vi "Transmit Command.vi"(8 "error in":errorcluster, 10 "Command":string, 11 "3300 in":refnum<class "3300.lvclass">) -> (0 "error out":errorcluster, 3 "3300 out":refnum<class "3300.lvclass">)   [LabVIEW 2019, in "3300.lvlib" / "3300.lvclass"]
uses:
  Library/3300.lvclass
  Library/3300.lvclass/3300.ctl
  <instrlib>/Agilent N330X Series/Agilent N330X Series.lvlib
  builds/Engine/Engine.lvlibp/Project/Engine.lvclass
  C:/Users/Public/Documents/Development/builds/Engine/Engine.lvlibp/Project/Engine.lvclass
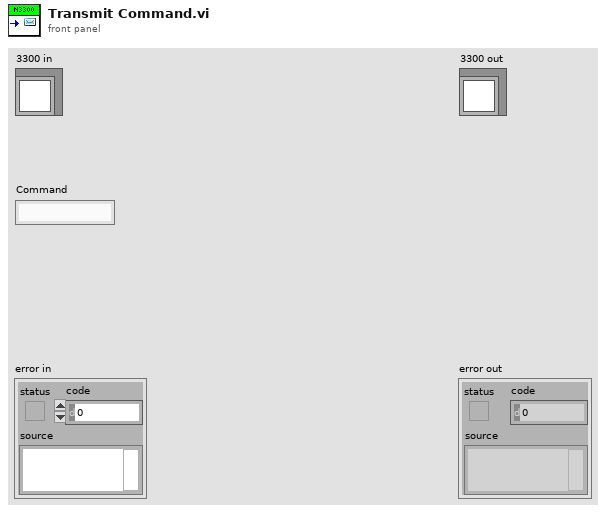
[diagram p1: front panel]
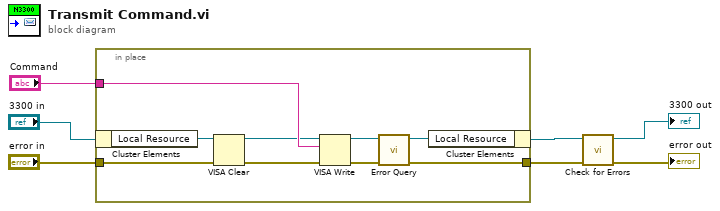
[diagram p0: block diagram]
diagram:
  n1 = in-place {
    in-place-border: "Command" -> [w15]
    in-place-border: "error in" -> [w8]
    in-place-border: [w11] -> w3
    n2 = in-place-cluster #1("3300 in") -> ("Local Resource"=w16:refnum<visa-resource-name>)
    n3 = VISA Clear(VISA resource name=w16, error in (no error)=w8) -> (VISA resource name out=w10:refnum<visa-resource-name>, error out=w9:errorcluster)
    n4 = VISA Write(VISA resource name=w10, write buffer=w15, error in (no error)=w9) -> (VISA resource name out=w14:refnum<visa-resource-name>, error out=w13:errorcluster)  [unwired: 1 out]
    n5 = call <instrlib>:"Error Query.vi"("error in (no error)"=w13, "VISA resource name"=w14) -> ("error out"=w11:errorcluster, "VISA resource name out"=w12:refnum<visa-resource-name>)  [unwired: 6 in, 2 out]
    n6 = in-place-cluster #1("Local Resource"=w12) -> (w4:refnum<class "3300.lvclass">)
  }
  n7 = call "Check for Errors.vi"("error in"=w3, "Engine in"=w4) -> ("error out"=→"error out":errorcluster, "Engine out"=→"3300 out":refnum<class "3300.lvclass">)  [unwired: 8 in]
